vi "Create 1D array of text and style.vi"(0 "Find tag ?":bool, 5 "Text duplicate":string, 7 "Style [ ]":T1[][](array[typedef]), 11 "error in (no error)":errorcluster) -> (8 "Style and text [ ]":T2(array[cluster]), 15 "error out":errorcluster)   [LabVIEW 2019]
doc: "Version 1.0\nDeveloped by Jean-Marc Simard\nCopyright © 2011, Exaprom Inc.\nAll rights reserved.\nLicense: BSD\n\nWith iTextSharp 4.1.6 (http://itextsharp.sourceforge.net)\nunder Mozilla Public License Version 1.1\n(http://www.mozilla.org/MPL/MPL-1.1.html)"
uses:
  <userlib>/Exaprom PDF/Controls/Text Controls/HTML tags.ctl
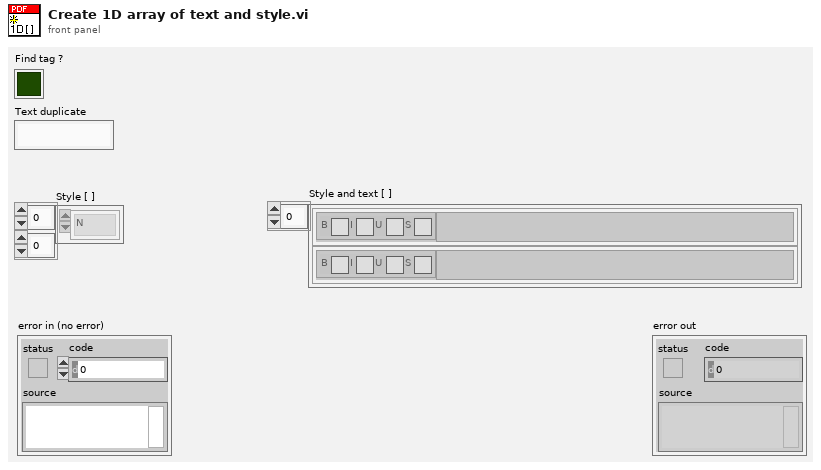
[diagram p1: front panel]
types:
  T1 = typedef "HTML tags.ctl" = enum16{"N", "b", "u", "s", "i"}
  T2 = cluster{"Style":cluster{"Bold":bool, "Italic":bool, "Underline":bool, "Strikeout":bool}, "Text 2":string}[]
  T3 = cluster{"Style":cluster{"Bold":bool, "Italic":bool, "Underline":bool, "Strikeout":bool}, "Text duplicate":string}
  T4 = cluster{"Bold":bool, "Italic":bool, "Underline":bool, "Strikeout":bool}
  T5 = cluster{"Style":cluster{"Bold":bool, "Italic":bool, "Underline":bool, "Strikeout":bool}, "Text duplicate":string}[]
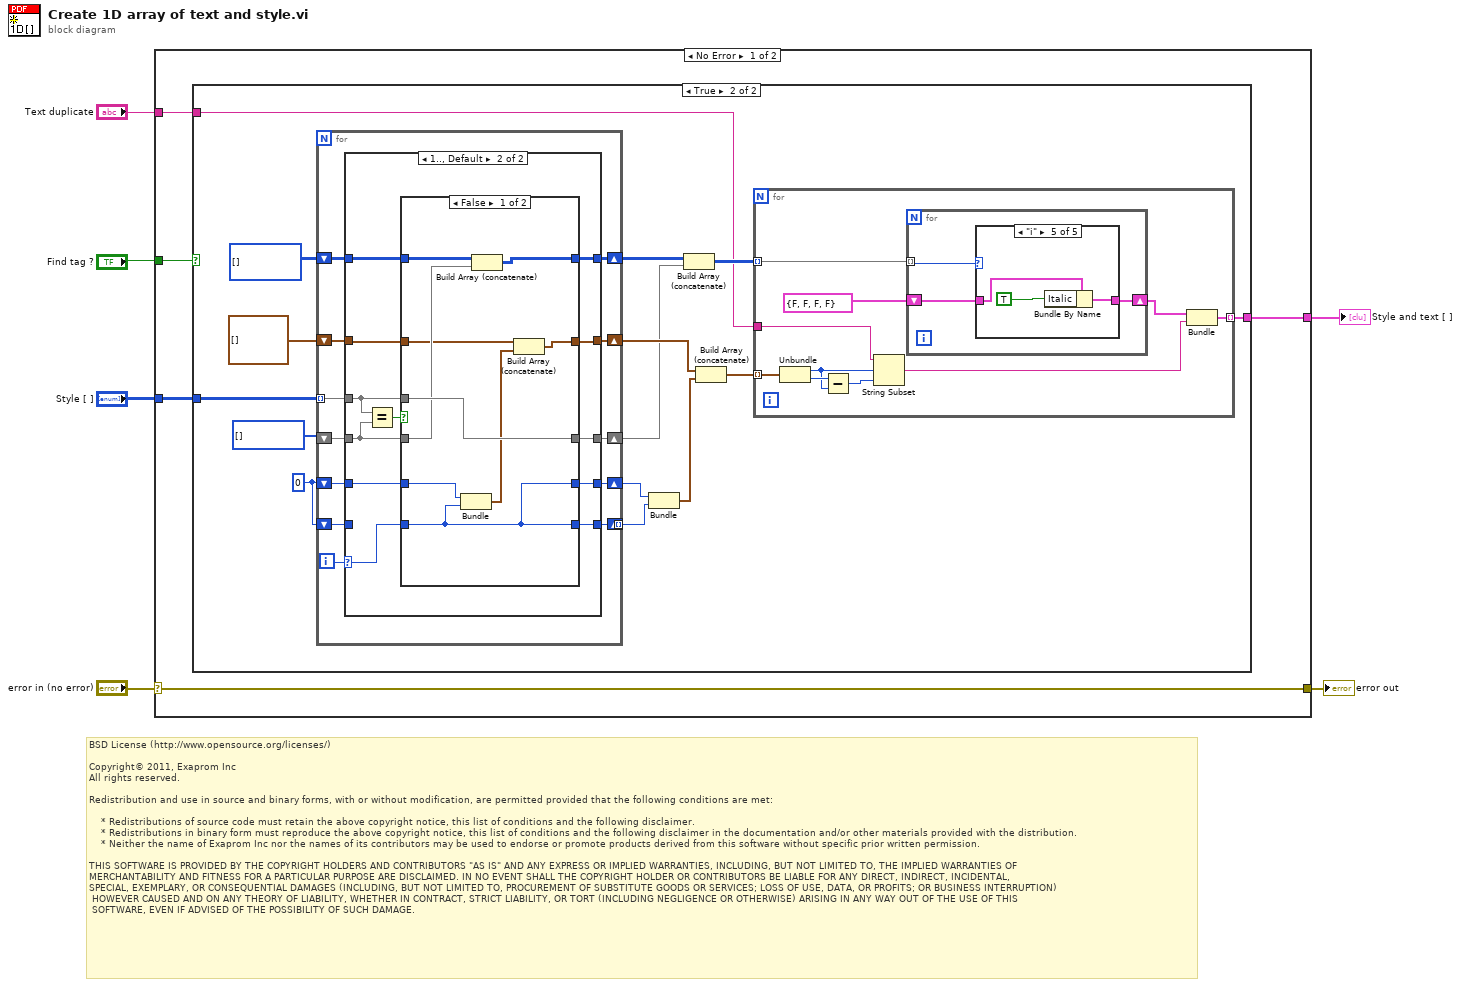
[diagram p0: block diagram]
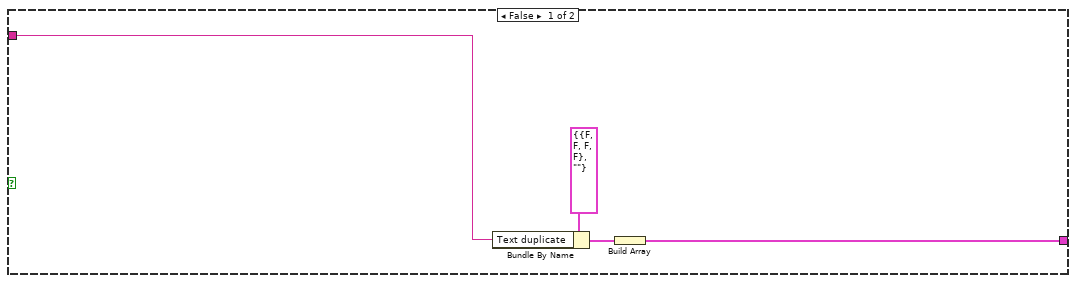
[diagram p2: hidden frame]
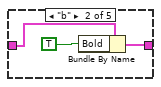
[diagram p4: hidden frame]
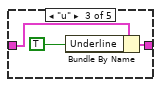
[diagram p5: hidden frame]
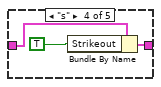
[diagram p6: hidden frame]
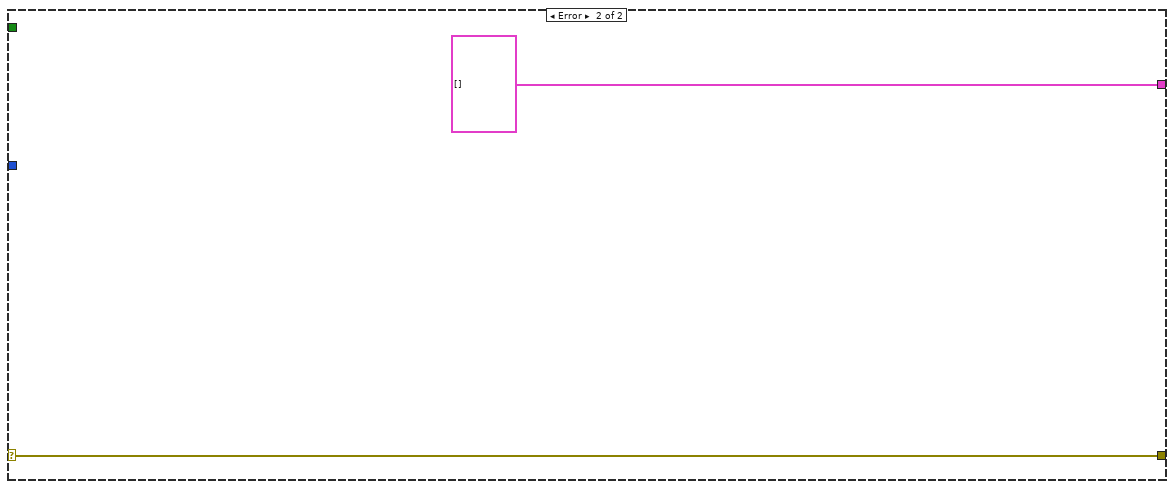
[diagram p9: hidden frame]
diagram:
  # "BSD License (http://www.opensource.org/licenses/)\n\nCopyright© 2011, Exaprom Inc\nAll rights reserved.\n\nRedistribution and use in source and binary forms, with or without modification, are permitted provided that the following conditions are met:\n\n    * Redistributions of source code must retain the above copyright notice, this list of conditions and the following disclaimer.\n    * Redistributions in binary form must reproduce the above copyright notice, this list of conditions and the following disclaimer in the documentation and/or other materials provided with the distribution.\n    * Neither the name of Exaprom Inc nor the names of its contributors may be used to endorse or promote products derived from this software without specific prior written permission.\n\nTHIS SOFTWARE IS PROVIDED BY THE COPYRIGHT HOLDERS AND CONTRIBUTORS \"AS IS\" AND ANY EXPRESS OR IMPLIED WARRANTIES, INCLUDING, BUT NOT LIMITED TO, THE IMPLIED WARRANTIES OF \nMERCHANTABILITY AND FITNESS FOR A PARTICULAR PURPOSE ARE DISCLAIMED. IN NO EVENT SHALL THE COPYRIGHT HOLDER OR CONTRIBUTORS BE LIABLE FOR ANY DIRECT, INDIRECT, INCIDENTAL,\nSPECIAL, EXEMPLARY, OR CONSEQUENTIAL DAMAGES (INCLUDING, BUT NOT LIMITED TO, PROCUREMENT OF SUBSTITUTE GOODS OR SERVICES; LOSS OF USE, DATA, OR PROFITS; OR BUSINESS INTERRUPTION)\n HOWEVER CAUSED AND ON ANY THEORY OF LIABILITY, WHETHER IN CONTRACT, STRICT LIABILITY, OR TORT (INCLUDING NEGLIGENCE OR OTHERWISE) ARISING IN ANY WAY OUT OF THE USE OF THIS\n SOFTWARE, EVEN IF ADVISED OF THE POSSIBILITY OF SUCH DAMAGE."
  n1 = case shown="No Error" "error in (no error)" {
    selector: "error in (no error)" -> [w11 w101]
    tunnel: [w11 w101] -> w6
    tunnel: [w10 T5 []] -> w4
    tunnel: "Style [ ]" -> [w9 _]
    tunnel: "Text duplicate" -> [w8 _]
    tunnel: "Find tag ?" -> [w7 _]
    frame No Error {
      n2 = case shown="True" w7 {
        tunnel: [w12 w18] -> w10
        tunnel: w9 -> [_ w17]
        tunnel: w8 -> [w14 w16]
        frame False {
          n3 = Bundle By Name(cluster=T3 {"Style"={"Bold"=FALSE, "Italic"=FALSE, "Underline"=FALSE, "Strikeout"=FALSE}, "Text duplicate"=""}, "Text duplicate"=w14) -> (w13:T3)
          n4 = Build Array(w13) -> (w12:T5)
        }
        frame True {
          w22 = 0
          w21 = T1[] [] items=["N", "b", "u", "s", "i"]
          w20 = T1[][] [] items=["N", "b", "u", "s", "i"]
          n5 = for {
            shift-right: [w63] -> w23
            shift-left: w20 -> [w58]
            shift-right: [w65] -> w25
            shift-left: cluster{i32, i32}[] [] -> [w64]
            tunnel: w17 -> [w66] mode=indexing
            shift-right: [w67] -> w24
            shift-left: w21 -> [w62]
            shift-right: [w61] -> w26
            shift-left: w22 -> [w60]
            shift-right: [w57] -> w28
            shift-left: w22 -> [w59]
            tunnel: [w57] -> _ mode=indexing
            i -> [w68]
            n6 = case shown="1.., Default" w68 {
              selector: w68 -> [_ w82]
              tunnel: [w72 w80] -> w67
              tunnel: w66 -> [w72 w74]
              tunnel: [w73 w76] -> w65
              tunnel: w64 -> [w73 w75]
              tunnel: [w69 w77] -> w63
              tunnel: w62 -> [_ w79]
              tunnel: [w71 w84] -> w61
              tunnel: w60 -> [w71 w83]
              tunnel: [w70 w81] -> w57
              tunnel: w59 -> [w70 _]
              tunnel: w58 -> [w69 w78]
              frame 0 {
              }
              frame 1.., Default {
                n7 = Equal?(x=w74, y=w79) -> (x = y?=w85:bool)
                n8 = case shown="False" w85 {
                  tunnel: [w86 w99] -> w84
                  tunnel: w83 -> [w93 w99]
                  tunnel: w82 -> [w86 w98]
                  tunnel: [w86 w98] -> w81
                  tunnel: [w94 w97] -> w80
                  tunnel: w79 -> [w91 w97]
                  tunnel: w74 -> [w94 _]
                  tunnel: w78 -> [w92 w96]
                  tunnel: [w90 w96] -> w77
                  tunnel: [w88 w95] -> w76
                  tunnel: w75 -> [w89 w95]
                  frame False {
                    n9 = Bundle(w93, w86) -> (w87:cluster{i32, i32})  [unwired: 1 out]
                    n10 = Build Array (concatenate)(w92, w91) -> (w90:T1[][])
                    n11 = Build Array (concatenate)(w89, w87) -> (w88:cluster{i32, i32}[])
                  }
                  frame True {
                  }
                }
              }
            }
          }
          n12 = Bundle(w26, w28) -> (w27:cluster{i32, i32})  [unwired: 1 out]
          n13 = Build Array (concatenate)(w23, w24) -> (w29:T1[][])
          n14 = Build Array (concatenate)(w25, w27) -> (w30:cluster{i32, i32}[])
          n15 = for {
            tunnel: w29 -> [w39] mode=indexing
            tunnel: w30 -> [w37] mode=indexing
            tunnel: w16 -> [w38]
            tunnel: [w32] -> w18 mode=indexing
            n16 = Unbundle(w37) -> (w35:i32, w36:i32)
            n17 = Subtract(x=w36, y=w35) -> (x-y=w34:i32)
            n18 = String Subset(string=w38, offset (0)=w35, length (rest)=w34) -> (substring=w31:string)
            n19 = for {
              shift-right: [w42] -> w33
              shift-left: T4 {"Bold"=FALSE, "Italic"=FALSE, "Underline"=FALSE, "Strikeout"=FALSE} ("Style") -> [w41]
              tunnel: w39 -> [w43] mode=indexing
              n20 = case shown="\"i\"" w43 {
                tunnel: [w44 w46 w49 w52 w55] -> w42
                tunnel: w41 -> [w44 w47 w50 w53 w56]
                frame "N", Default {
                }
                frame "b" {
                  n21 = Bundle By Name(cluster=w47, "Bold"=TRUE) -> (w46:T4)
                }
                frame "u" {
                  n22 = Bundle By Name(cluster=w50, "Underline"=TRUE ("Bold")) -> (w49:T4)
                }
                frame "s" {
                  n23 = Bundle By Name(cluster=w53, "Strikeout"=TRUE ("Bold")) -> (w52:T4)
                }
                frame "i" {
                  n24 = Bundle By Name(cluster=w56, "Italic"=TRUE ("Bold")) -> (w55:T4)
                }
              }
            }
            n25 = Bundle("Style"=w33, "Text duplicate"=w31) -> (w32:T3)  [unwired: 1 out]
          }
        }
      }
    }
    frame Error {
    }
  }
  "error out" <- w6
  "Style and text [ ]" <- w4
